vi "1629_Side E1.vi"(8 "error in (no error)":errorcluster, 9 "1629_E1 inputs":T8={"1629 side E Ref ROI before transformation"={"Global Rectangle"=[], "Contours"=[]}, "Ref Search Direction"=2, "Ref Edge Options"={"Edge Polarity"=2, "Kernel Size"=3, "Width"=3, "Minimum Edge Strength"=50.0, "Interpolation Type"=enum."Zero Order", "Data Processing Method"=enum."Average"}, "Ref Line Options"={"Number of Lines"=1, "Type"=enum."Best Edge Rake", "Min. Score"=10.0, "Max. Score"=1000.0, "Orientation"=0.0, "Angle Range"=10.0, "Angle Tolerance"=1.0, "Step Size"=3, "Min. SNR (db)"=0.0, "Min. Points (%)"=25.0, "Hough Iterations"=5}, "Meas ROI-1 Descriptor before transformation"={"Global Rectangle"=[], "Contours"=[]}, "Meas-1 Step Size"=5, "Meas-1 Scan Direction"=2, "Meas-1 Edge Options"={"Edge Polarity"=0, "Kernel Size"=3, "Width"=3, "Minimum Edge Strength"=50.0, "Interpolation Type"=enum."Zero Order", "Data Processing Method"=enum."Average"}, "Meas ROI-2 Descriptor Before Transformation"={"Global Rectangle"=[], "Contours"=[]}, "Meas-2 Scan Direction"=0, "Meas-2 Edge Options"={"Edge Polarity"=2, "Kernel Size"=3, "Width"=3, "Minimum Edge Strength"=50.0, "Interpolation Type"=enum."Zero Order", "Data Processing Method"=enum."Average"}, "Meas-2 Line Options"={"Number of Lines"=1, "Type"=enum."Best Edge Rake", "Min. Score"=10.0, "Max. Score"=1000.0, "Orientation"=0.0, "Angle Range"=10.0, "Angle Tolerance"=1.0, "Step Size"=3, "Min. SNR (db)"=0.0, "Min. Points (%)"=25.0, "Hough Iterations"=5}, "Ellipse Center"={"X"=0.0, "Y"=0.0}} {"Meas-2 Line Options"."Min. Points (%)" min=0.0 max=100.0; "Meas-2 Line Options"."Min. SNR (db)" min=0.0; "Meas-2 Line Options"."Max. Score" min=0.0 max=1024.0; "Meas-2 Line Options"."Min. Score" min=0.0 max=1024.0 step=1.0; "Meas-2 Edge Options"."Edge Polarity" items=["All Edges", "Rising Edges", "Falling Edges"]; "Meas-2 Edge Options"."Minimum Edge Strength" format="%.2f"; "Meas-2 Edge Options"."Width" step=2; "Meas-2 Edge Options"."Kernel Size" step=2; "Meas-2 Scan Direction" items=["Left to Right", "Right to Left", "Top to Bottom", "Bottom to Top"]; "Meas ROI-2 Descriptor Before Transformation"."Contours"."Type" items=["No Selection", "Point", "Line", "Rectangle", "Oval", "Polygon", "Freehand Region", "Annulus", "Unused2", "Unused3", "Broken Line", "Freehand Line", "Rotated Rectangle"]; "Meas-1 Edge Options"."Edge Polarity" items=["All Edges", "Rising Edges", "Falling Edges"]; "Meas-1 Edge Options"."Minimum Edge Strength" format="%.2f"; "Meas-1 Edge Options"."Width" step=2; "Meas-1 Edge Options"."Kernel Size" step=2; "Meas-1 Scan Direction" items=["Left To Right", "Right To Left", "Top To Bottom", "Bottom To Top"]; "Meas ROI-1 Descriptor before transformation"."Contours"."Type" items=["No Selection", "Point", "Line", "Rectangle", "Oval", "Polygon", "Freehand Region", "Annulus", "Unused2", "Unused3", "Broken Line", "Freehand Line", "Rotated Rectangle"]; "Ref Line Options"."Min. Points (%)" min=0.0 max=100.0; "Ref Line Options"."Min. SNR (db)" min=0.0; "Ref Line Options"."Max. Score" min=0.0 max=1024.0; "Ref Line Options"."Min. Score" min=0.0 max=1024.0 step=1.0; "Ref Edge Options"."Edge Polarity" items=["All Edges", "Rising Edges", "Falling Edges"]; "Ref Edge Options"."Minimum Edge Strength" format="%.2f"; "Ref Edge Options"."Width" step=2; "Ref Edge Options"."Kernel Size" step=2; "Ref Search Direction" items=["Left to Right", "Right to Left", "Top to Bottom", "Bottom to Top"]; "1629 side E Ref ROI before transformation"."Contours"."Type" items=["No Selection", "Point", "Line", "Rectangle", "Oval", "Polygon", "Freehand Region", "Annulus", "Unused2", "Unused3", "Broken Line", "Freehand Line", "Rotated Rectangle"]}, 10 "Calibrated Image":T1, 11 "Input Image":T1(plugin-control)) -> (0 "error out":errorcluster, 1 "1629_E1 outtput":T2, 3 "Image Out":T1)   [LabVIEW 2019, in "Algorithm.lvclass"]
uses:
  FrameworkOverrides/Algorithm.lvclass
  <vilib>/vision/NI_Vision_Development_Module.lvlib
  <vilib>/vision/Measure.llb/Edge Polarity.ctl
  <vilib>/vision/Measure.llb/Edge Options.ctl
  <vilib>/vision/Measure.llb/Straight Edge Process.ctl
  <vilib>/vision/Measure.llb/Straight Edge Options.ctl
  <vilib>/vision/Image Controls.llb/IMAQ Image.ctl
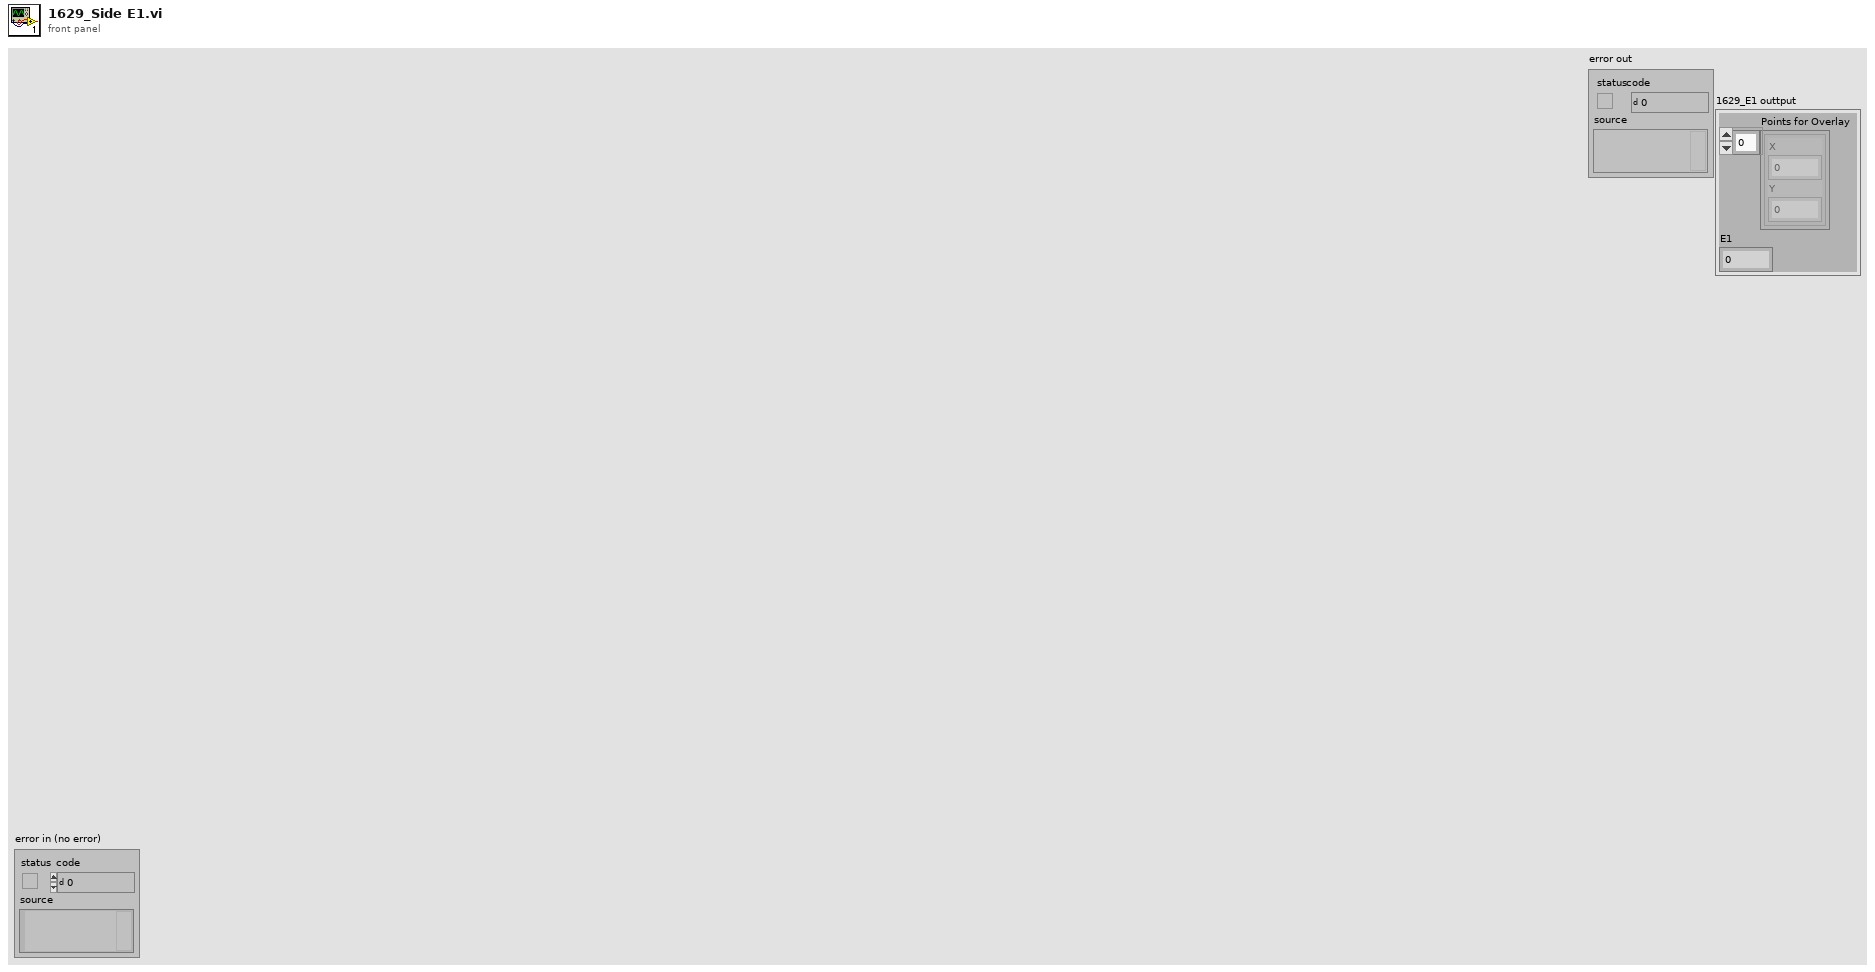
[diagram p1: front panel]
types:
  T1 = typedef "IMAQ Image.ctl" = refnum<image>
  T2 = cluster{"Points for Overlay":cluster{"X":sgl, "Y":sgl}[], "E1":sgl}
  T3 = typedef "ROI Descriptor" = cluster{"Global Rectangle":i32[], "Contours":cluster{"ID":enum32{"External", "Internal"}, "Type":u32, "Coordinates":i32[]}[]}
  T4 = typedef "Edge Options.ctl" = cluster{"Edge Polarity":T5, "Kernel Size":u32, "Width":u32, "Minimum Edge Strength":sgl, "Interpolation Type":enum32{"Zero Order", "Bilinear", "Quadratic", "Cubic", "Bilinear Fixed"}, "Data Processing Method":enum32{"Average", "Median"}}
  T5 = typedef "Edge Polarity.ctl" = u32
  T6 = typedef "Straight Edge Options.ctl" = cluster{"Number of Lines":i32, "Type":T7, "Min. Score":dbl, "Max. Score":dbl, "Orientation":dbl, "Angle Range":dbl, "Angle Tolerance":dbl, "Step Size":u32, "Min. SNR (db)":dbl, "Min. Points (%)":dbl, "Hough Iterations":i32}
  T7 = typedef "Straight Edge Process.ctl" = enum32{"First Edge Rake", "Best Edge Rake", "Hough Edge Rake", "First Edge Projection", "Best Edge Projection"}
  T8 = cluster{"1629 side E Ref ROI before transformation":T3, "Ref Search Direction":u32, "Ref Edge Options":T4, "Ref Line Options":T6, "Meas ROI-1 Descriptor before transformation":T3, "Meas-1 Step Size":u32, "Meas-1 Scan Direction":u16, "Meas-1 Edge Options":T4, "Meas ROI-2 Descriptor Before Transformation":T3, "Meas-2 Scan Direction":u32, "Meas-2 Edge Options":T4, "Meas-2 Line Options":T6, "Ellipse Center":cluster{"X":sgl, "Y":sgl}}
  T9 = cluster{"Points for Overlay":cluster{"X":sgl, "Y":sgl}[], "element":sgl}
  T10 = cluster{"Point 1":cluster{"X":sgl, "Y":sgl}, "Point 2":cluster{"X":sgl, "Y":sgl}}
  T11 = enum16{"Get First Edge", "Get First + Last Edge", "Get All Edges", "Get Best Edge"}
  T12 = typedef "IMAQ Rectangle" = cluster{"Left":i32, "Top":i32, "Right":i32, "Bottom":i32, "Rotation":dbl}
  T13 = cluster{"ID":enum32{"External", "Internal"}, "Type":u32, "Coordinates":i32[]}[]
  T14 = cluster{"ID":enum32{"External", "Internal"}, "Type":u32, "Coordinates":i32[]}
  T15 = cluster{"Point1 (Pixels)":cluster{"X":sgl, "Y":sgl}, "Point2 (Pixels)":cluster{"X":sgl, "Y":sgl}, "Point1 (Real-World)":cluster{"X":sgl, "Y":sgl}, "Point2 (Real-World)":cluster{"X":sgl, "Y":sgl}, "Angle (Pixel)":dbl, "Angle (Real-World)":dbl, "Score":dbl, "Straightness":dbl, "Average SNR (db)":dbl, "Calibration Valid":bool}[]
  T16 = cluster{"Straight Edges[0]":cluster{"Point1 (Pixels)":cluster{"X":sgl, "Y":sgl}, "Point2 (Pixels)":cluster{"X":sgl, "Y":sgl}, "Point1 (Real-World)":cluster{"X":sgl, "Y":sgl}, "Point2 (Real-World)":cluster{"X":sgl, "Y":sgl}, "Angle (Pixel)":dbl, "Angle (Real-World)":dbl, "Score":dbl, "Straightness":dbl, "Average SNR (db)":dbl, "Calibration Valid":bool}, "Straight Edges[1]":cluster{"Point1 (Pixels)":cluster{"X":sgl, "Y":sgl}, "Point2 (Pixels)":cluster{"X":sgl, "Y":sgl}, "Point1 (Real-World)":cluster{"X":sgl, "Y":sgl}, "Point2 (Real-World)":cluster{"X":sgl, "Y":sgl}, "Angle (Pixel)":dbl, "Angle (Real-World)":dbl, "Score":dbl, "Straightness":dbl, "Average SNR (db)":dbl, "Calibration Valid":bool}, "Straight Edges[2]":cluster{"Point1 (Pixels)":cluster{"X":sgl, "Y":sgl}, "Point2 (Pixels)":cluster{"X":sgl, "Y":sgl}, "Point1 (Real-World)":cluster{"X":sgl, "Y":sgl}, "Point2 (Real-World)":cluster{"X":sgl, "Y":sgl}, "Angle (Pixel)":dbl, "Angle (Real-World)":dbl, "Score":dbl, "Straightness":dbl, "Average SNR (db)":dbl, "Calibration Valid":bool}, "Straight Edges[3]":cluster{"Point1 (Pixels)":cluster{"X":sgl, "Y":sgl}, "Point2 (Pixels)":cluster{"X":sgl, "Y":sgl}, "Point1 (Real-World)":cluster{"X":sgl, "Y":sgl}, "Point2 (Real-World)":cluster{"X":sgl, "Y":sgl}, "Angle (Pixel)":dbl, "Angle (Real-World)":dbl, "Score":dbl, "Straightness":dbl, "Average SNR (db)":dbl, "Calibration Valid":bool}, "Straight Edges[4]":cluster{"Point1 (Pixels)":cluster{"X":sgl, "Y":sgl}, "Point2 (Pixels)":cluster{"X":sgl, "Y":sgl}, "Point1 (Real-World)":cluster{"X":sgl, "Y":sgl}, "Point2 (Real-World)":cluster{"X":sgl, "Y":sgl}, "Angle (Pixel)":dbl, "Angle (Real-World)":dbl, "Score":dbl, "Straightness":dbl, "Average SNR (db)":dbl, "Calibration Valid":bool}, "Straight Edges[5]":cluster{"Point1 (Pixels)":cluster{"X":sgl, "Y":sgl}, "Point2 (Pixels)":cluster{"X":sgl, "Y":sgl}, "Point1 (Real-World)":cluster{"X":sgl, "Y":sgl}, "Point2 (Real-World)":cluster{"X":sgl, "Y":sgl}, "Angle (Pixel)":dbl, "Angle (Real-World)":dbl, "Score":dbl, "Straightness":dbl, "Average SNR (db)":dbl, "Calibration Valid":bool}, "Straight Edges[6]":cluster{"Point1 (Pixels)":cluster{"X":sgl, "Y":sgl}, "Point2 (Pixels)":cluster{"X":sgl, "Y":sgl}, "Point1 (Real-World)":cluster{"X":sgl, "Y":sgl}, "Point2 (Real-World)":cluster{"X":sgl, "Y":sgl}, "Angle (Pixel)":dbl, "Angle (Real-World)":dbl, "Score":dbl, "Straightness":dbl, "Average SNR (db)":dbl, "Calibration Valid":bool}, "Straight Edges[7]":cluster{"Point1 (Pixels)":cluster{"X":sgl, "Y":sgl}, "Point2 (Pixels)":cluster{"X":sgl, "Y":sgl}, "Point1 (Real-World)":cluster{"X":sgl, "Y":sgl}, "Point2 (Real-World)":cluster{"X":sgl, "Y":sgl}, "Angle (Pixel)":dbl, "Angle (Real-World)":dbl, "Score":dbl, "Straightness":dbl, "Average SNR (db)":dbl, "Calibration Valid":bool}, "Straight Edges[8]":cluster{"Point1 (Pixels)":cluster{"X":sgl, "Y":sgl}, "Point2 (Pixels)":cluster{"X":sgl, "Y":sgl}, "Point1 (Real-World)":cluster{"X":sgl, "Y":sgl}, "Point2 (Real-World)":cluster{"X":sgl, "Y":sgl}, "Angle (Pixel)":dbl, "Angle (Real-World)":dbl, "Score":dbl, "Straightness":dbl, "Average SNR (db)":dbl, "Calibration Valid":bool}}
  T17 = cluster{"Point1 (Pixels)":cluster{"X":sgl, "Y":sgl}, "Point2 (Pixels)":cluster{"X":sgl, "Y":sgl}, "Point1 (Real-World)":cluster{"X":sgl, "Y":sgl}, "Point2 (Real-World)":cluster{"X":sgl, "Y":sgl}, "Angle (Pixel)":dbl, "Angle (Real-World)":dbl, "Score":dbl, "Straightness":dbl, "Average SNR (db)":dbl, "Calibration Valid":bool}
  T18 = typedef "Edge New.ctl" = cluster{"Location (Pixel)":cluster{"X":sgl, "Y":sgl}, "Location (Real-World)":cluster{"X":sgl, "Y":sgl}, "Distance (Pixel)":dbl, "Distance (Real-World)":dbl, "Strength":dbl, "Noise":dbl, "Rising?":bool}
  T19 = typedef "Search Line.ctl" = cluster{"Start Point":cluster{"X":sgl, "Y":sgl}, "End Point":cluster{"X":sgl, "Y":sgl}, "Edge Info":T18[], "Edge Map":dbl[], "Calibration Valid":bool}
  T20 = cluster{"Location (Pixel)":cluster{"X":sgl, "Y":sgl}, "Start Point":cluster{"X":sgl, "Y":sgl}}
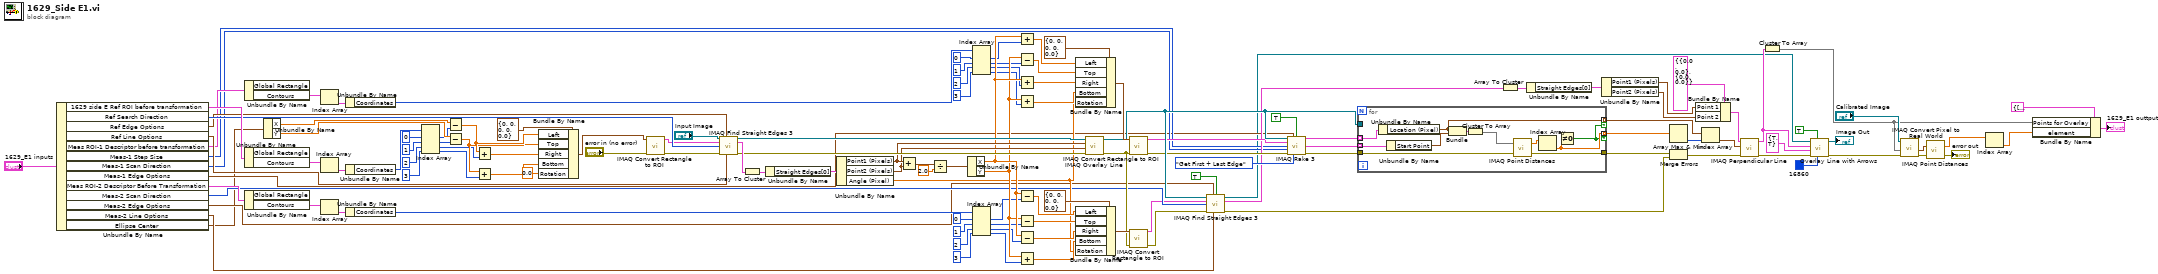
[diagram p0: block diagram]
diagram:
  n1 = Unbundle By Name("1629_E1 inputs") -> ("1629 side E Ref ROI before transformation"=w31:T3, "Ref Search Direction"=w30:u32, "Ref Edge Options"=w29:T4, "Ref Line Options"=w28:T6, "Meas ROI-1 Descriptor before transformation"=w27:T3, "Meas-1 Step Size"=w26:u32, "Meas-1 Scan Direction"=w25:u16, "Meas-1 Edge Options"=w24:T4, "Meas ROI-2 Descriptor Before Transformation"=w23:T3, "Meas-2 Scan Direction"=w22:u32, "Meas-2 Edge Options"=w21:T4, "Meas-2 Line Options"=w20:T6, "Ellipse Center"=w19:cluster{"X":sgl, "Y":sgl})
  n2 = Unbundle By Name(w27) -> ("Contours"=w67:T13)  [unwired: 1 out]
  n3 = Unbundle By Name(w31) -> ("Contours"=w37:T13)  [unwired: 1 out]
  n4 = Unbundle By Name(w23) -> ("Contours"=w49:T13)  [unwired: 1 out]
  n5 = Unbundle By Name(w19) -> ("X"=w128:sgl, "Y"=w126:sgl)
  n6 = Index Array(array=w67) -> (element=w66:T14)  [unwired: 1 in]
  n7 = Index Array(array=w37) -> (element=w38:T14)  [unwired: 1 in]
  n8 = Index Array(array=w49) -> (element=w50:T14)  [unwired: 1 in]
  n9 = Unbundle By Name(w66) -> ("Coordinates"=w65:i32[])
  n10 = Unbundle By Name(w38) -> ("Coordinates"=w39:i32[])
  n11 = Unbundle By Name(w50) -> ("Coordinates"=w51:i32[])
  n12 = Index Array(array=w39, index #1=0 ("index"), index #2=1 ("index"), index #3=2 ("index"), index #4=3 ("index")) -> (element #1=w36:i32, element #2=w35:i32, element #3=w34:i32, element #4=w33:i32)
  n13 = Subtract(x=w128, y=w36) -> (x-y=w124:sgl)
  n14 = Subtract(x=w126, y=w35) -> (x-y=w122:sgl)
  n15 = Add(x=w124, y=w34) -> (x+y=w123:sgl)
  n16 = Add(x=w122, y=w33) -> (x+y=w121:sgl)
  n17 = Bundle By Name(cluster=T12 {"Left"=0, "Top"=0, "Right"=0, "Bottom"=0, "Rotation"=0.0} ("Rectangle"), "Left"=w124, "Top"=w122, "Right"=w123, "Bottom"=w121, "Rotation"=0.0) -> (w125:T12)
  n18 = call "IMAQ Convert Rectangle to ROI"("error in (no error)"="error in (no error)", "Rectangle"=w125) -> ("error out"=w115:errorcluster, "ROI Descriptor"=w1:T3)  [unwired: 7 in]
  n19 = call "IMAQ Find Straight Edges 3"("Image"="Input Image", "Edge Options"=w29, "ROI Descriptor"=w1, "Search Direction"=w30, "error in (no error)"=w115, "Line Options"=w28) -> ("Image (duplicate)"=w116:T1, "Straight Edges"=w118:T15, "error out"=w114:errorcluster)  [unwired: 5 in, 2 out]
  n20 = Array To Cluster(array=w118) -> (cluster=w117:T16)
  n21 = Unbundle By Name(w117) -> ("Straight Edges[0]"=w119:T17)
  n22 = Unbundle By Name(w119) -> ("Point1 (Pixels)"=w112:cluster{"X":sgl, "Y":sgl}, "Point2 (Pixels)"=w111:cluster{"X":sgl, "Y":sgl}, "Angle (Pixel)"=w92:dbl)
  n23 = Add(x=w112, y=w111) -> (x+y=w110:cluster{"X":sgl, "Y":sgl})
  n24 = Divide(x=w110, y=2.0) -> (x/y=w109:cluster{"X":dbl, "Y":dbl})
  n25 = Unbundle By Name(w109) -> ("X"=w97:dbl, "Y"=w94:dbl)
  n26 = Index Array(array=w65, index #1=0 ("index"), index #2=1 ("index"), index #3=2 ("index"), index #4=3 ("index")) -> (element #1=w60:i32, element #2=w59:i32, element #3=w58:i32, element #4=w57:i32)
  n27 = Index Array(array=w51, index #1=0 ("index"), index #2=1 ("index"), index #3=2 ("index"), index #4=3 ("index")) -> (element #1=w48:i32, element #2=w47:i32, element #3=w46:i32, element #4=w45:i32)
  n28 = Add(x=w97, y=w60) -> (x+y=w106:dbl)
  n29 = Subtract(x=w94, y=w59) -> (x-y=w105:dbl)
  n30 = Add(x=w97, y=w58) -> (x+y=w104:dbl)
  n31 = Add(x=w94, y=w57) -> (x+y=w103:dbl)
  n32 = Subtract(x=w97, y=w48) -> (x-y=w98:dbl)
  n33 = Subtract(x=w94, y=w47) -> (x-y=w95:dbl)
  n34 = Subtract(x=w97, y=w46) -> (x-y=w96:dbl)
  n35 = Add(x=w94, y=w45) -> (x+y=w93:dbl)
  n36 = Bundle By Name(cluster=T12 {"Left"=0, "Top"=0, "Right"=0, "Bottom"=0, "Rotation"=0.0} ("Rectangle"), "Left"=w106, "Top"=w105, "Right"=w104, "Bottom"=w103, "Rotation"=w92) -> (w108:T12)
  n37 = Bundle By Name(cluster=T12 {"Left"=0, "Top"=0, "Right"=0, "Bottom"=0, "Rotation"=0.0} ("Rectangle"), "Left"=w98, "Top"=w95, "Right"=w96, "Bottom"=w93, "Rotation"=w92) -> (w101:T12)
  n38 = call "IMAQ Overlay Line"("error in (no error)"=w114, "End Point"=w111, "Start Point"=w112, "Image"=w116) -> ("error out"=w99:errorcluster, "Image Out"=w100:T1)  [unwired: 6 in]
  n39 = call "IMAQ Convert Rectangle to ROI"("error in (no error)"=w99, "Rectangle"=w108) -> ("error out"=w90:errorcluster, "ROI Descriptor"=w91:T3)  [unwired: 7 in]
  n40 = call "IMAQ Convert Rectangle to ROI"("error in (no error)"=w99, "Rectangle"=w101) -> ("error out"=w83:errorcluster, "ROI Descriptor"=w4:T3)  [unwired: 7 in]
  n41 = call "IMAQ Find Straight Edges 3"("Image"=w100, "Edge Options"=w21, "Optimized Mode"=TRUE, "ROI Descriptor"=w4, "Search Direction"=w22, "error in (no error)"=w83, "Line Options"=w20) -> ("Image (duplicate)"=w3:T1, "Straight Edges"=w82:T15, "error out"=w79:errorcluster)  [unwired: 4 in, 2 out]
  n42 = call "IMAQ Rake 3"("Image"=w100, "Edge Options"=w24, "Optimized Mode"=TRUE, "ROI Descriptor"=w91, "Step Size"=w26, "Scan Direction"=w25, "error in (no error)"=w90, "Process"=T11."Get First + Last Edge") -> ("First Edges"=w87:T18[], "Search Lines"=w88:T19[], "error out"=w73:errorcluster)  [unwired: 4 in, 1 out]
  n43 = for {
    tunnel: w88 -> [w139] mode=indexing
    tunnel: w100 -> [_]
    tunnel: w87 -> [w138] mode=indexing
    tunnel: [w136] -> w86 mode=indexing if=w135
    tunnel: [w132] -> w85 mode=indexing if=w135
    tunnel: [w133] -> w72
    tunnel: w73 -> [w134]
    n44 = Unbundle By Name(w138) -> ("Location (Pixel)"=w132:cluster{"X":sgl, "Y":sgl})
    n45 = Unbundle By Name(w139) -> ("Start Point"=w131:cluster{"X":sgl, "Y":sgl})
    n46 = Bundle("Location (Pixel)"=w132, "Start Point"=w131) -> (w130:T20)  [unwired: 1 in]
    n47 = Cluster To Array(cluster=w130) -> (array=w129:cluster{"X":sgl, "Y":sgl}[])
    n48 = call "IMAQ Point Distances"("Points"=w129, "error in (no error)"=w134) -> ("Distances"=w137:sgl[], "error out"=w133:errorcluster)  [unwired: 3 in]
    n49 = Index Array(array=w137) -> (element=w136:sgl)  [unwired: 1 in]
    n50 = Not Equal To 0?(x=w136) -> (x != 0?=w135:bool)
  }
  n51 = Array To Cluster(array=w82) -> (cluster=w81:T16)
  n52 = Unbundle By Name(w81) -> ("Straight Edges[0]"=w80:T17)
  n53 = Unbundle By Name(w80) -> ("Point1 (Pixels)"=w76:cluster{"X":sgl, "Y":sgl}, "Point2 (Pixels)"=w75:cluster{"X":sgl, "Y":sgl})
  n54 = Array Max & Min(array=w86) -> (min index (indices)=w84:i32)  [unwired: 3 out]
  n55 = Merge Errors(w72, w79) -> (w71:errorcluster)
  n56 = Bundle By Name(cluster=T10 {"Point 1"={"X"=0.0, "Y"=0.0}, "Point 2"={"X"=0.0, "Y"=0.0}} ("Line"), "Point 1"=w76, "Point 2"=w75) -> (w74:T10)
  n57 = Index Array(array=w85, index=w84) -> (element=w78:cluster{"X":sgl, "Y":sgl})
  n58 = call "IMAQ Perpendicular Line"("error in (no error)"=w71, "Point"=w78, "Line"=w74) -> ("error out"=w12:errorcluster, "Perpendicular Line"=w18:T10)  [unwired: 6 in, 1 out]
  n59 = Cluster To Array(cluster=w18) -> (array=w9:cluster{"X":sgl, "Y":sgl}[])
  n60 = call <vilib>:"Overlay Line with Arrows.vi"("Color"=u32 16860, "Draw line?"=TRUE, "error in (no error)"=w12, "Arrows"=cluster{"Start point":bool, "End point":bool} {"Start point"=TRUE, "End point"=TRUE}, "Line Coordinates"=w18, "Image In"=w3) -> ("error out"=w11:errorcluster, "Image Out"=→"Image Out":T1)  [unwired: 4 out]
  n61 = call "IMAQ Convert Pixel to Real World"("error in (no error)"=w11, "Array of Pixel Coordinates"=w9, "Calibrated Image"="Calibrated Image") -> ("error out"=w14:errorcluster, "Array of Real World Coordinates"=w16:cluster{"X":sgl, "Y":sgl}[])  [unwired: 3 in, 4 out]
  n62 = call "IMAQ Point Distances"("Points"=w16, "error in (no error)"=w14) -> ("Distances"=w15:sgl[], "error out"=→"error out":errorcluster)  [unwired: 3 in]
  n63 = Index Array(array=w15) -> (element=w8:sgl)  [unwired: 1 in]
  n64 = Bundle By Name(cluster=T9 {"Points for Overlay"=[], "element"=0.0}, "Points for Overlay"=w9, "element"=w8) -> (→"1629_E1 outtput":T9)
